vi "Write Multiple Holding Registers.vi"(7 "unit ID":u8, 8 "error in":errorcluster, 9 "registers to write":u16[](array[numeric]), 10 "starting address":u16, 11 "Modbus slave in":refnum<class "Modbus Slave.lvclass">) -> (0 "error out":errorcluster, 3 "Modbus slave out":refnum<class "Modbus Slave.lvclass">)   [LabVIEW 2013, in "Modbus Library - Advance.lvlib" / "Modbus Slave.lvclass"]
doc: "Writes <B>registers to write</B> starting at <B>starting address</B> to the device holding registers."
uses:
  Modbus Slave.lvclass
  Modbus Slave.lvclass/Modbus Slave.ctl
  Standard Data Model/Standard Data Model.lvclass
  Super Data Model/Super Data Model.lvclass
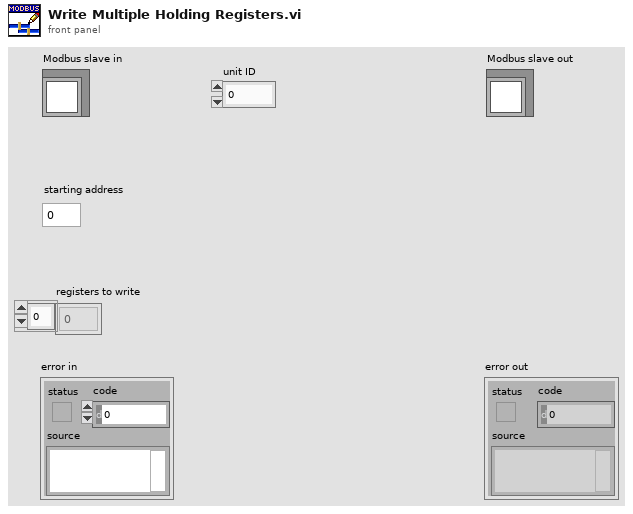
[diagram p1: front panel]
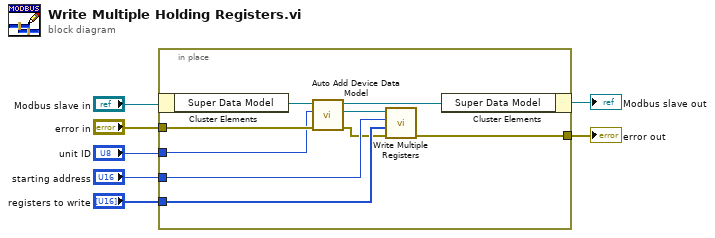
[diagram p0: block diagram]
diagram:
  n1 = in-place {
    in-place-border: "registers to write" -> [w10]
    in-place-border: "starting address" -> [w11]
    in-place-border: [w8] -> w1
    in-place-border: "error in" -> [w15]
    in-place-border: "unit ID" -> [w13]
    n2 = in-place-cluster #1("Modbus slave in") -> ("Super Data Model"=w16:refnum<class "Super Data Model.lvclass">)
    n3 = call "Auto Add Device Data Model.vi"("error in"=w15, "unit ID"=w13, "Super Data Model in"=w16) -> ("error out"=w9:errorcluster, "device data model"=w12:refnum<class "Standard Data Model.lvclass">, "Super Data Model out"=w14:refnum<class "Super Data Model.lvclass">)  [unwired: 6 in]
    n4 = call-dynamic "Write Multiple Registers.vi"("error in"=w9, "register values"=w10, "starting address"=w11, "device data model in"=w12) -> ("error out"=w8:errorcluster)  [unwired: 6 in, 1 out]
    n5 = in-place-cluster #1("Super Data Model"=w14) -> (→"Modbus slave out":refnum<class "Modbus Slave.lvclass">)
  }
  "error out" <- w1
